vi "Obtain Message Queue.vi"(8 "error in (no error)":errorcluster, 11 "Queue Name":string) -> (0 "error out":errorcluster, 3 "queue out":refnum<queue>)   [LabVIEW 2023, in "HAF.lvlib"]
doc: "Creates a new Message Queue with the Message Structure used by the Framework."
uses:
  HAF.lvlib
  Message.ctl
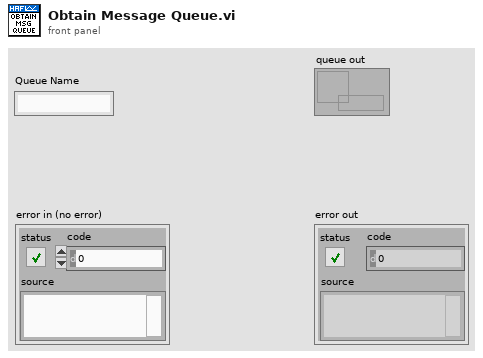
[diagram p1: front panel]
types:
  T1 = typedef "HAF.lvlib/Message.ctl" = cluster{"Message Id":string, "Message Data":variant}
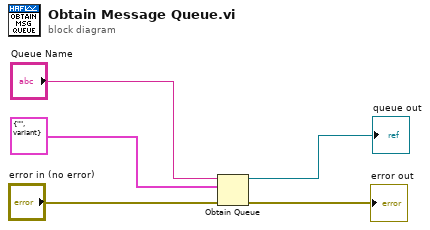
[diagram p0: block diagram]
diagram:
  n1 = Obtain Queue(name (unnamed)="Queue Name", element data type=T1 {"Message Id"="", "Message Data"=variant} ("Message Structure"), error in (no error)="error in (no error)") -> (queue out=→"queue out":refnum<queue>, error out=→"error out":errorcluster)  [unwired: 2 in, 1 out]
